vi "SPC_get_init_status.vi"(8 "Error In":errorcluster, 9 "No of Usable\nModules":i32, 10 "Module No":i16 min=0 max=7 step=1, 11 "DLL Path":path) -> (0 "Error Out":errorcluster, 2 "Module No":i16, 3 "DLL Path":path, 4 "Message":string="Init not done", 5 "Init Status code":i16=-1)   [LabVIEW 2023]
doc: "The procedure returns the initialisation result code set by the function SPC_init. The possible \nvalues are shown below (see also spcm_def.h):\nINIT_ SPC_OK 0 no error\nINIT_ SPC_NOT_DONE -1 init not done\nINIT_ SPC_WRONG_EEP_CHKSUM -2 wrong EEPROM checksum \nINIT_ SPC_WRONG_MOD_ID -3 wrong module identification code\nINIT_ SPC_HARD_TEST_ERR -4 hardware test failed\nINIT_ SPC_CANT_OPEN_PCI_CARD -5 cannot open PCI card\nINIT_ SPC_MOD_IN_USE -6 module in use (locked) - cannot initialise\nINIT_ SPC_WINDRVR_VER -7 incorrect WinDriver version\nINIT_ SPC_WRONG_LICENSE -8 corrupted license key\nINIT_SPC_FIRMWARE_VER -9 incorrect firmware version of DPC/SPC module\nINIT_SPC_NO_LICENSE -10 license key not read from registry\nINIT_SPC_LICENSE_NOT_VALID -11 license is not valid for SPCM DLL\nINIT_SPC_LICENSE_DATE_EXP -12 license date expired\nINIT_SPC_XILINX_ERR -1xx Xilinx chip configuration error - where xx = Xilinx error code\n\ninfo@becker-hickl.com"
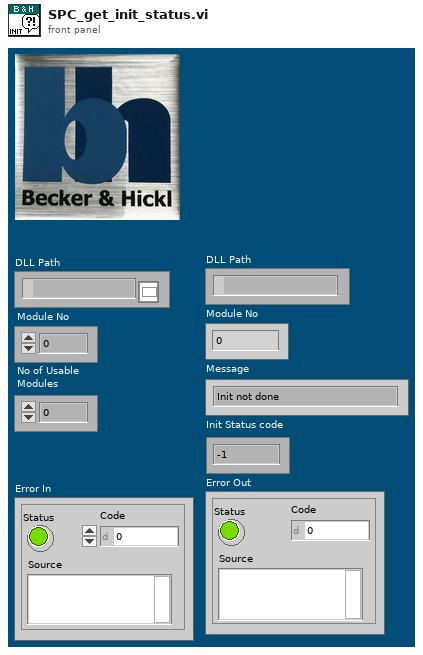
[diagram p1: front panel]
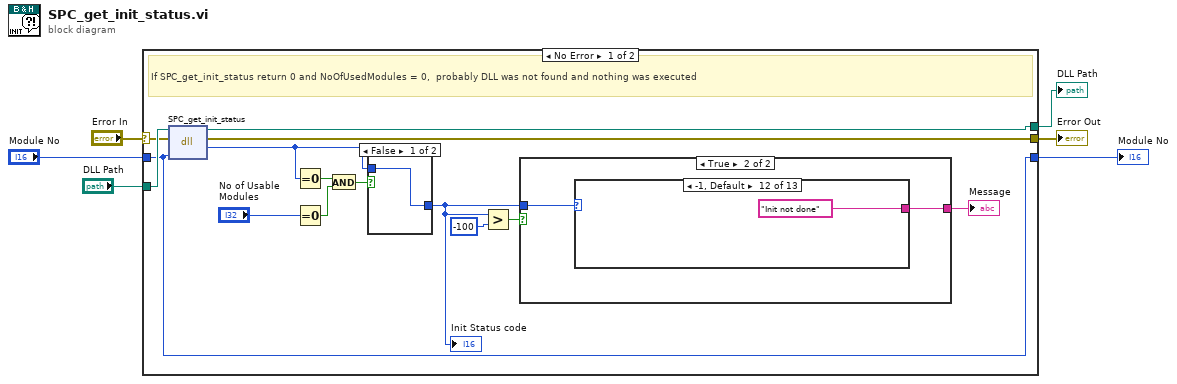
[diagram p0: block diagram]
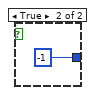
[diagram p2: hidden frame]
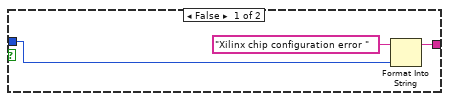
[diagram p3: hidden frame]
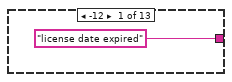
[diagram p4: hidden frame]
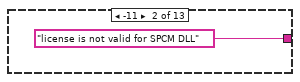
[diagram p5: hidden frame]
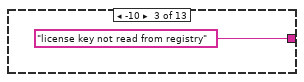
[diagram p6: hidden frame]
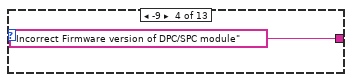
[diagram p7: hidden frame]
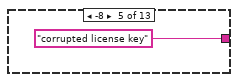
[diagram p8: hidden frame]
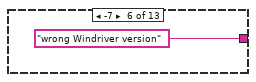
[diagram p9: hidden frame]
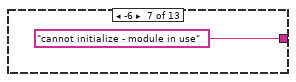
[diagram p10: hidden frame]
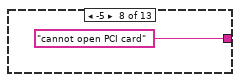
[diagram p11: hidden frame]
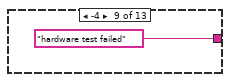
[diagram p12: hidden frame]
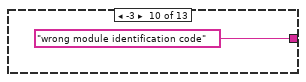
[diagram p13: hidden frame]
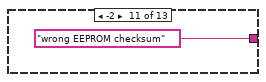
[diagram p14: hidden frame]
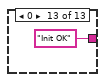
[diagram p15: hidden frame]
diagram:
  n1 = case shown="No Error" "Error In" {
    selector: "Error In" -> [w11 w43]
    tunnel: "DLL Path" -> [w12 w42]
    tunnel: [w10 w43] -> w5
    tunnel: [w9 w42] -> w4
    tunnel: "Module No" -> [w7 w41]
    tunnel: [w7 w41] -> w1
    frame No Error {
      # "If SPC_get_init_status return 0 and NoOfUsedModules = 0,  probably DLL was not found and nothing was executed"
      n2 = dll-call lib="D:/spcm/lib/lab_view/lv10.0/spcm32.dll" fn="SPC_get_init_status"(path in=w12, error in=w11, "mod_no"=w7) -> (path out=w9:path, error out=w10:errorcluster, "return type"=w13:i16)  [unwired: 2 in]
      n3 = Equal To 0?(x=w13) -> (x = 0?=w17:bool)
      n4 = Equal To 0?(x="No of Usable\nModules") -> (x = 0?=w16:bool)
      n5 = And(x=w17, y=w16) -> (x .and. y?=w15:bool)
      n6 = case shown="False" w15 {
        tunnel: [w21 i16 -1] -> w14
        tunnel: w13 -> [w21 _]
        frame False {
        }
        frame True {
        }
      }
      "Init Status code" <- w14
      n7 = Greater?(x=w14, y=i16 -100) -> (0:w19:bool)
      n8 = case shown="True" w19 {
        tunnel: w14 -> [w25 w27]
        tunnel: [w24 w26] -> w20
        frame False {
          n9 = Format Into String(initial string="Xilinx chip configuration error ", w25) -> (resulting string=w24:string)  [unwired: 2 in, 1 out]
        }
        frame True {
          n10 = case shown="-1, Default" w27 {
            tunnel: ["license date expired" "license is not valid for SPCM DLL" "license key not read from registry" "Incorrect Firmware version of DPC/SPC module" "corrupted license key" "wrong Windriver version" "cannot initialize - module in use" "cannot open PCI card" "hardware test failed" "wrong module identification code" "wrong EEPROM checksum" "Init not done" "Init OK"] -> w26
            frame -12 {
            }
            frame -11 {
            }
            frame -10 {
            }
            frame -9 {
            }
            frame -8 {
            }
            frame -7 {
            }
            frame -6 {
            }
            frame -5 {
            }
            frame -4 {
            }
            frame -3 {
            }
            frame -2 {
            }
            frame -1, Default {
            }
            frame 0 {
            }
          }
        }
      }
      "Message" <- w20
    }
    frame Error {
    }
  }
  "DLL Path" <- w4
  "Error Out" <- w5
  "Module No" <- w1
